vi "Write Spreadsheet.vi"(8 "error in (no error)":errorcluster, 11 "Excel Legacy in":refnum<class "Excel Legacy.lvclass">) -> (0 "error out":errorcluster, 3 "Excel Legacy out":refnum<class "Excel Legacy.lvclass">)   [LabVIEW 2013, in "Excel Legacy.lvclass"]
uses:
  Excel Legacy.lvclass
  Spreadsheet.lvclass
  Excel Legacy.lvclass/Excel Legacy.ctl
  C:/PhaeronGit/LVNPOI/Resources/NPOI 2.1.1 dotnet2/NPOI.dll
  Resources/NPOI 2.1.1 dotnet2/NPOI.dll
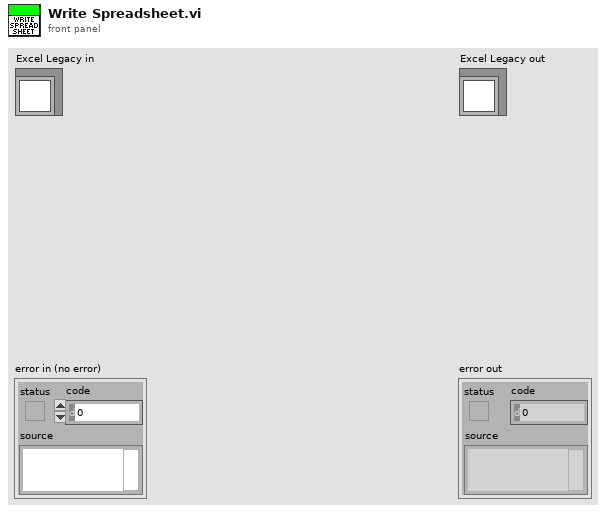
[diagram p1: front panel]
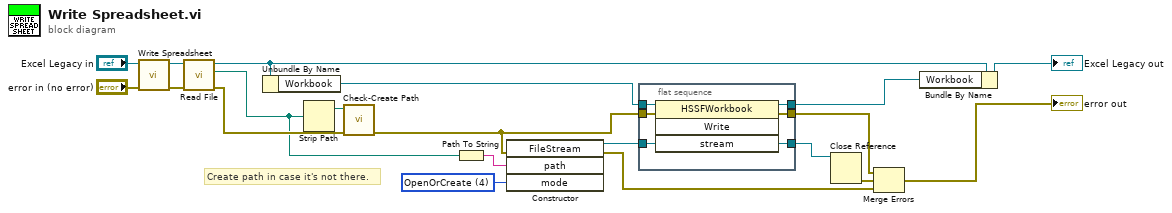
[diagram p0: block diagram]
diagram:
  w9 = 4 items=["CreateNew"=1, "Create"=2, "Open"=3, "OpenOrCreate"=4, "Truncate"=5, "Append"=6] ("mode")
  # "Create path in case it's not there."
  n1 = call-parent "Write Spreadsheet.vi"("error in (no error)"="error in (no error)", "Spreadsheet in"="Excel Legacy in") -> ("error out"=w17:errorcluster, "Spreadsheet out"=w18:refnum<class "Excel Legacy.lvclass">)  [unwired: 8 in]
  n2 = call-dynamic "Read File.vi"("error in (no error)"=w17, "Spreadsheet in"=w18) -> ("error out"=w7:errorcluster, "File"=w3:path, "Spreadsheet out"=w5:refnum<class "Excel Legacy.lvclass">)  [unwired: 7 in]
  n3 = Unbundle By Name(w5) -> ("Workbook"=w4:refnum<k24>)
  n4 = Strip Path(path=w3) -> (stripped path=w16:path)  [unwired: 1 out]
  n5 = call <vilib>:"Check-Create Path.vi"("error in"=w7, "Path"=w16) -> ("error out"=w15:errorcluster)  [unwired: 8 in, 1 out]
  n6 = Path To String(path=w3) -> (string=w8:string)
  n7 = constructor class="FileStream"(error in=w15, "path"=w8, "mode"=w9) -> (reference out=w10:refnum<k24>, error out=w14:errorcluster)  [unwired: 2 in, 3 out]
  n8 = flat-sequence {
    tunnel: w4 -> [w25]
    tunnel: [w24] -> w1
    tunnel: w15 -> [w23]
    tunnel: w10 -> [w21]
    tunnel: [w22] -> w11
    tunnel: [w21] -> w13
    frame #0 {
      n9 = invoke class="HSSFWorkbook" method="Write"(reference=w25, error in=w23, "stream"=w21) -> (reference out=w24:refnum<k24>, error out=w22:errorcluster)  [unwired: 1 in, 2 out]
    }
  }
  n10 = Close Reference(reference=w13) -> (error out=w12:errorcluster)  [unwired: 1 in]
  n11 = Merge Errors(w11, w12, w14) -> (→"error out":errorcluster)
  n12 = Bundle By Name(cluster=w5, "Workbook"=w1) -> (→"Excel Legacy out":refnum<class "Excel Legacy.lvclass">)
